vi "_Publish DP Indicators(VI).vi"(7 "VIRef(Caller VI)/RefMgr":refnum<vi>, 8 "error in (no error)":errorcluster, 9 "force update(F)":bool, 11 "SILAPI In":T1) -> (0 "error out":errorcluster, 1 "Binded DPs":string[](array[string]), 3 "SILAPI Out":T1)   [LabVIEW 2017, in "TagDB RefManager.lvlib"]
uses:
  TagDB RefManager.lvlib
  <userlib>/_NEVSTOP/TagDB/Typedef/TagDB.ctl
  10d0bc68-ff5b-4b3e-94b6-72122e87f5c0.vi
  936e1e9c-d5b6-4b4e-ad99-7c7dab878fa3.vi
  12cc79ca-27a7-4410-b99e-89b61dace636.vi
  99199be5-3273-4500-92d5-279e96ad7927.vi
  <userlib>/_NEVSTOP/TagDB/_Support/DataAccess/_NameCacher.vi
  <userlib>/_NEVSTOP/TagDB/_Support/Error/_[error50002]Invalid DataType.vi
  <userlib>/_NEVSTOP/TagDB/_Support/Error/_[error50000]Invalid DB REF.vi
  <userlib>/_NEVSTOP/TagDB/_Support/DataAccess/TagDB Ref to DVR.vi
  <userlib>/_NEVSTOP/TagDB/_Support/URL/TRIM-BOTH-SPACE.vi
  <userlib>/_NEVSTOP/TagDB/_Support/Error/_Build Error Cluster.vi
  <userlib>/_NEVSTOP/TagDB/TagDB.lvlib
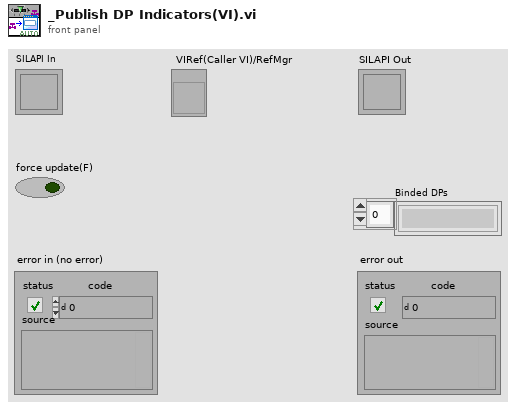
[diagram p1: front panel]
types:
  T1 = typedef "TagDB.lvlib/TagDB.ctl" = refnum<k1>
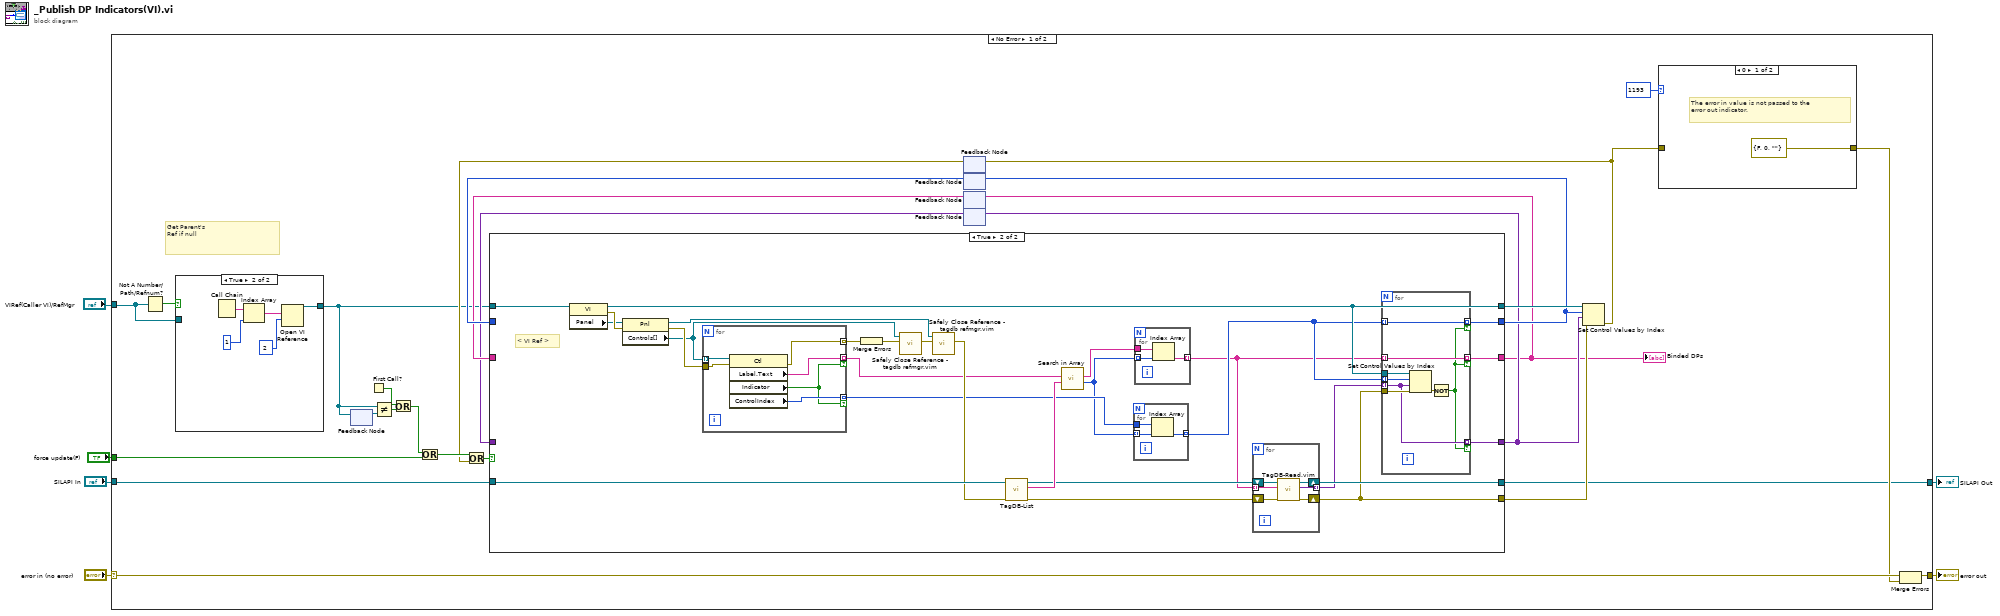
[diagram p0: block diagram]
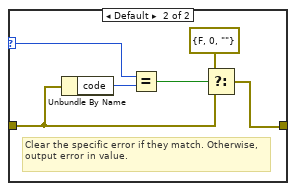
[diagram p3: hidden frame]
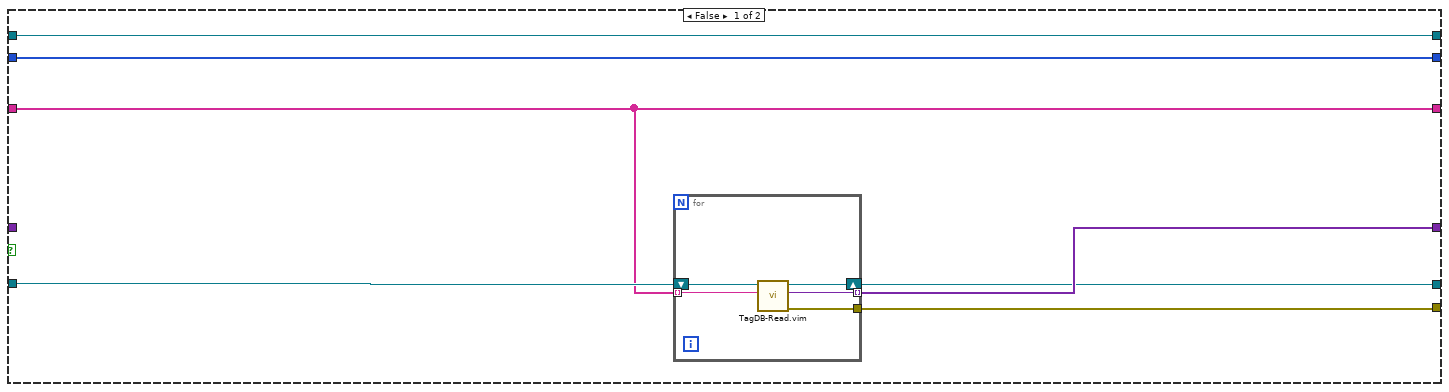
[diagram p4: hidden frame]
diagram:
  n1 = case shown="No Error" "error in (no error)" {
    selector: "error in (no error)" -> [w26 w111]
    tunnel: "force update(F)" -> [w32 _]
    tunnel: [w27 w111] -> w5
    tunnel: "SILAPI In" -> [w24 w112]
    tunnel: "VIRef(Caller VI)/RefMgr" -> [w12 _]
    tunnel: [w14 w112] -> w1
    frame No Error {
      # "Get Parent's\nRef if null"
      n2 = Not A Number/Path/Refnum?(number/path/refnum=w12) -> (NaN/Path/Refnum?=w13:bool)
      n3 = case shown="True" w13 {
        tunnel: [w33 w34] -> w8
        tunnel: w12 -> [w33 _]
        frame False {
        }
        frame True {
          n4 = Call Chain() -> (call chain=w38:string[])
          n5 = Index Array(array=w38, index=1 ("Index")) -> (element=w36:string)
          n6 = Open VI Reference(vi path=w36, options=2) -> (vi reference=w34:refnum<vi>)  [unwired: 4 in, 1 out]
        }
      }
      n7 = feedback #1() -> (w11:refnum<vi>)  [unwired: 1 in]
      n8 = feedback-in #1(w8) -> ()
      n9 = First Call?() -> (First Call?: T/F=w9:bool)
      n10 = Not Equal?(x=w8, y=w11) -> (x != y?=w10:bool)
      n11 = Or(x=w9, y=w10) -> (x .or. y?=w7:bool)
      n12 = Or(x=w7, y=w32) -> (x .or. y?=w28:bool)
      n13 = feedback #2() -> (w16:errorcluster)  [unwired: 1 in]
      n14 = Or(x=w28, y=w16) -> (x .or. y?=w18:bool)
      n15 = feedback #3() -> (w29:i32[])  [unwired: 1 in]
      n16 = feedback #4() -> (w25:string[])  [unwired: 1 in]
      n17 = feedback #5() -> (w21:variant[])  [unwired: 1 in]
      n18 = case shown="True" w18 {
        tunnel: [w52 w73] -> w31
        tunnel: w8 -> [w52 w84]
        tunnel: [w51 w77] -> w30
        tunnel: w29 -> [w51 _]
        tunnel: [w49 w78] -> w19
        tunnel: w25 -> [w49 _]
        tunnel: [w47 w76] -> w22
        tunnel: w24 -> [w50 w83]
        tunnel: [w48 w79] -> w23
        tunnel: w21 -> [_ _]
        tunnel: [w46 w81] -> w14
        frame False {
          n19 = for {
            tunnel: w49 -> [w56] mode=indexing
            tunnel: [w55] -> w48
            tunnel: [w54] -> w47 mode=indexing
            shift-right: [w53] -> w46
            shift-left: w50 -> [w57]
            n20 = call "TagDB-Read.vim"("name"=w56, "TagDB"=w57) -> ("error out"=w55:errorcluster, "Value"=w54:variant, "TagDB(dup)"=w53:T1)  [unwired: 4 in, 3 out]
          }
        }
        frame True {
          # "< VI Ref >"
          n21 = property class="VI"(reference=w84) -> (reference out=w73:refnum<vi>, error out=w75:errorcluster, "Panel"=w74:refnum<vi>)  [unwired: 1 in]
          n22 = property class="Pnl"(reference=w74, error in=w75) -> (reference out=w65:refnum<vi>, error out=w71:errorcluster, "Controls[]"=w66:refnum<vi>[])
          n23 = for {
            tunnel: w66 -> [w102] mode=indexing
            tunnel: [w101] -> w60 mode=indexing if=w99
            tunnel: [w100] -> w63 mode=indexing if=w99
            tunnel: [w98] -> w72 mode=indexing
            tunnel: w71 -> [w97]
            n24 = property class="Ctl"(reference=w102, error in=w97) -> (error out=w98:errorcluster, "Label.Text"=w101:string, "Indicator"=w99:bool, "ControlIndex"=w100:i32)  [unwired: 1 out]
          }
          n25 = Merge Errors(w72) -> (w67:errorcluster)
          n26 = call "Safely Close Reference - tagdb refmgr.vim"("error in (no error)"=w67, "Reference"=w66) -> ("error out"=w68:errorcluster)  [unwired: 9 in]
          n27 = call "Safely Close Reference - tagdb refmgr.vim"("error in (no error)"=w68, "Reference"=w65) -> ("error out"=w64:errorcluster)  [unwired: 9 in]
          n28 = call <userlib>:"TagDB-List.vi"("error in (no error)"=w64, "TagDB"=w83) -> ("error out"=w82:errorcluster, "names"=w70:string[], "TagDB(dup)"=w69:T1)  [unwired: 6 in, 1 out]
          n29 = call "Search in Array.vi"("items to filter"=w70, "array"=w60) -> ("item Indexs"=w61:i32[], "array(dup)"=w58:string[])  [unwired: 4 in]
          n30 = for {
            tunnel: w61 -> [w90] mode=indexing
            tunnel: w63 -> [w89]
            tunnel: [w88] -> w62 mode=indexing
            n31 = Index Array(array=w89, index=w90) -> (element=w88:i32)
          }
          n32 = for {
            tunnel: w61 -> [w87] mode=indexing
            tunnel: w58 -> [w86]
            tunnel: [w85] -> w59 mode=indexing
            n33 = Index Array(array=w86, index=w87) -> (element=w85:string)
          }
          n34 = for {
            tunnel: [w94] -> w80 mode=indexing
            tunnel: w59 -> [w92] mode=indexing
            shift-right: [w93] -> w79
            shift-left: w82 -> [w96]
            shift-right: [w95] -> w81
            shift-left: w69 -> [w91]
            n35 = call "TagDB-Read.vim"("error in (no error)"=w96, "name"=w92, "TagDB"=w91) -> ("error out"=w93:errorcluster, "Value"=w94:variant, "TagDB(dup)"=w95:T1)  [unwired: 3 in, 3 out]
          }
          n36 = for {
            tunnel: w73 -> [w110]
            tunnel: w62 -> [w109] mode=indexing
            tunnel: w80 -> [w105] mode=indexing
            tunnel: w79 -> [w108]
            tunnel: [w107] -> w78 mode=indexing if=w103
            tunnel: w59 -> [w107] mode=indexing
            tunnel: [w106] -> w77 mode=indexing if=w103
            tunnel: w62 -> [w106] mode=indexing
            tunnel: [w105] -> w76 mode=indexing if=w103
            n37 = Set Control Values by Index(0:w110, 1:w109, 2:w105, 3:w108) -> (11:w104:errorcluster)
            n38 = Not(x=w104) -> (.not. x?=w103:bool)
          }
        }
      }
      "Binded DPs" <- w19
      n39 = feedback-in #3(w30) -> ()
      n40 = feedback-in #4(w19) -> ()
      n41 = feedback-in #5(w22) -> ()
      n42 = Set Control Values by Index(0:w31, 1:w30, 2:w22, 3:w23) -> (11:w17:errorcluster)
      n43 = feedback-in #2(w17) -> ()
      n44 = case shown="0" 1193 ("specific error code to clear (0: all)") {
        selector: 1193 ("specific error code to clear (0: all)") -> [_ w44]
        tunnel: w17 -> [_ w43]
        tunnel: [errorcluster {"status"=FALSE, "code"=0, "source"=""} ("error constant") w40] -> w20
        frame 0 {
          # "The error in value is not passed to the\nerror out indicator."
        }
        frame Default {
          # "Clear the specific error if they match. Otherwise, output error in value."
          n45 = Unbundle By Name(w43) -> ("code"=w45:i32)
          n46 = Equal?(x=w44, y=w45) -> (x = y?=w41:bool)
          n47 = Select(t=errorcluster {"status"=FALSE, "code"=0, "source"=""} ("error constant"), s=w41, f=w43) -> (s? t:f=w40:errorcluster)
        }
      }
      n48 = Merge Errors(w26, w20) -> (w27:errorcluster)
    }
    frame Error {
    }
  }
  "error out" <- w5
  "SILAPI Out" <- w1
